vi "IPI_PassorFail_static.vi"(11 "Static":T1) -> (0 "Fail":dbl, 1 "Pass":dbl, 2 "Fail":string, 3 "Pass":string)   [LabVIEW 2015]
panel:
  out "x/y":dbl
  out "数字":dbl
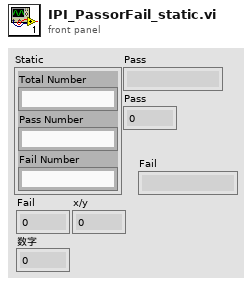
[diagram p1: front panel]
types:
  T1 = cluster{"Total Number":string, "Pass Number":string, "Fail Number":string}
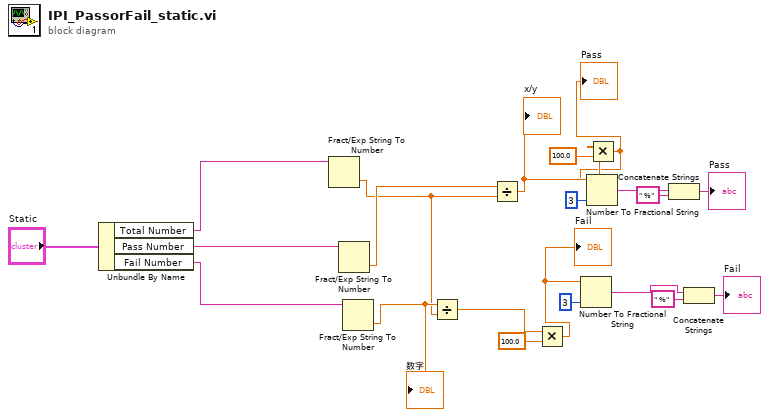
[diagram p0: block diagram]
diagram:
  n1 = Unbundle By Name("Static") -> ("Total Number"=w20:string, "Pass Number"=w19:string, "Fail Number"=w18:string)
  n2 = Fract/Exp String To Number(string=w20) -> (number=w15:dbl)  [unwired: 3 in, 1 out]
  n3 = Fract/Exp String To Number(string=w19) -> (number=w17:dbl)  [unwired: 3 in, 1 out]
  n4 = Fract/Exp String To Number(string=w18) -> (number=w16:dbl)  [unwired: 3 in, 1 out]
  "数字" <- w16
  n5 = Divide(x=w16, y=w15) -> (x/y=w2:dbl)
  n6 = Divide(x=w17, y=w15) -> (x/y=w6:dbl)
  "x/y" <- w6
  n7 = Multiply(x=w2, y=100.0) -> (x*y=w1:dbl)
  "Fail" <- w1
  n8 = Number To Fractional String(number=w1, precision (6)=i16 3 ("精度(6)")) -> (F-format string=w7:string)  [unwired: 2 in]
  n9 = Multiply(x=w6, y=100.0) -> (x*y=w4:dbl)
  "Pass" <- w4
  n10 = Number To Fractional String(number=w4, precision (6)=i16 3 ("精度(6)")) -> (F-format string=w12:string)  [unwired: 2 in]
  n11 = Concatenate Strings(w12, " %" ("字符串")) -> (→"Pass":string)
  n12 = Concatenate Strings(w7, " %" ("字符串")) -> (→"Fail":string)
